vi "Calibration Utility.vi"() -> ()   [LabVIEW 2019]
panel:
  in  "Tab 1":enum32{"Page 1", "Page 2"}(tab)
  in  "Main Tab":T1(tab)
  in  "Tab 2":enum32{"Page 1", "Page 2"}(tab)
  out "Title":string="Calibration Utility, vBETA1"
  out "Date":string="2/21/2012"
  out "Time":string="2:11:48 PM"
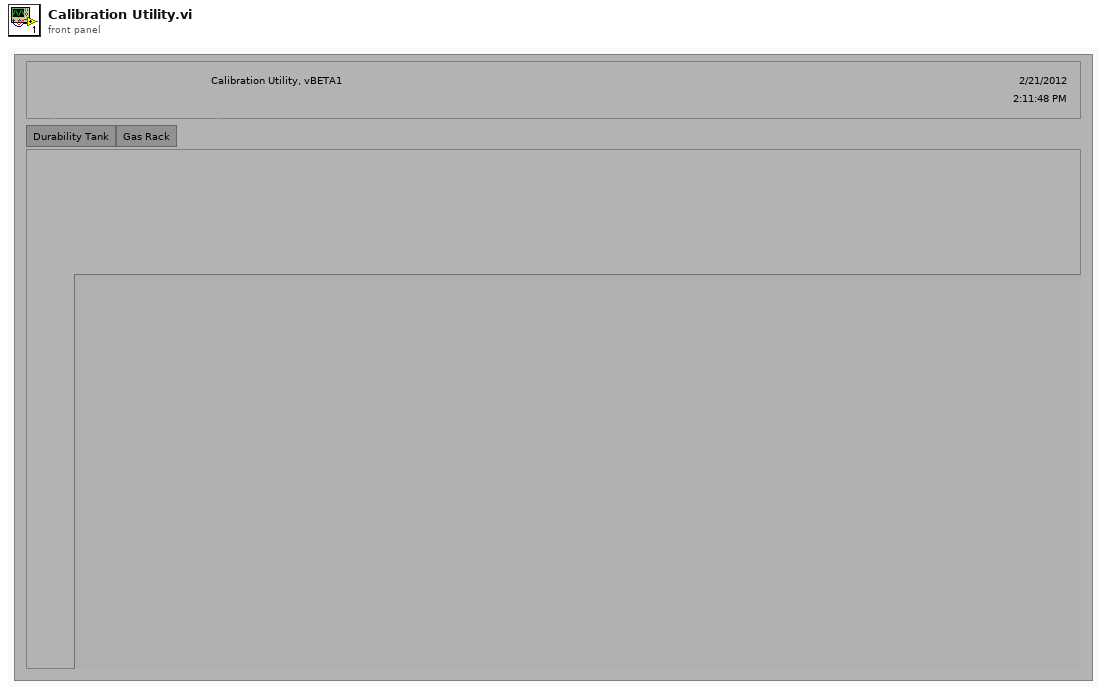
[diagram p1: front panel]
types:
  T1 = enum32{"Netway", "Durability Tank", "Gas Rack", "Dunk Tank"}
  T2 = enum32{"Page Enabled", "Page Disabled", "Page Disabled & Grayed"}
  T3 = enum32{"Invalid", "Standard", "Closed", "Hidden", "Minimized", "Maximized"}
  T4 = enum32{"invalid app kind", "Development System", "Run Time System", "Student Edition", "Embedded LabVIEW", "Evaluation", "Custom"}
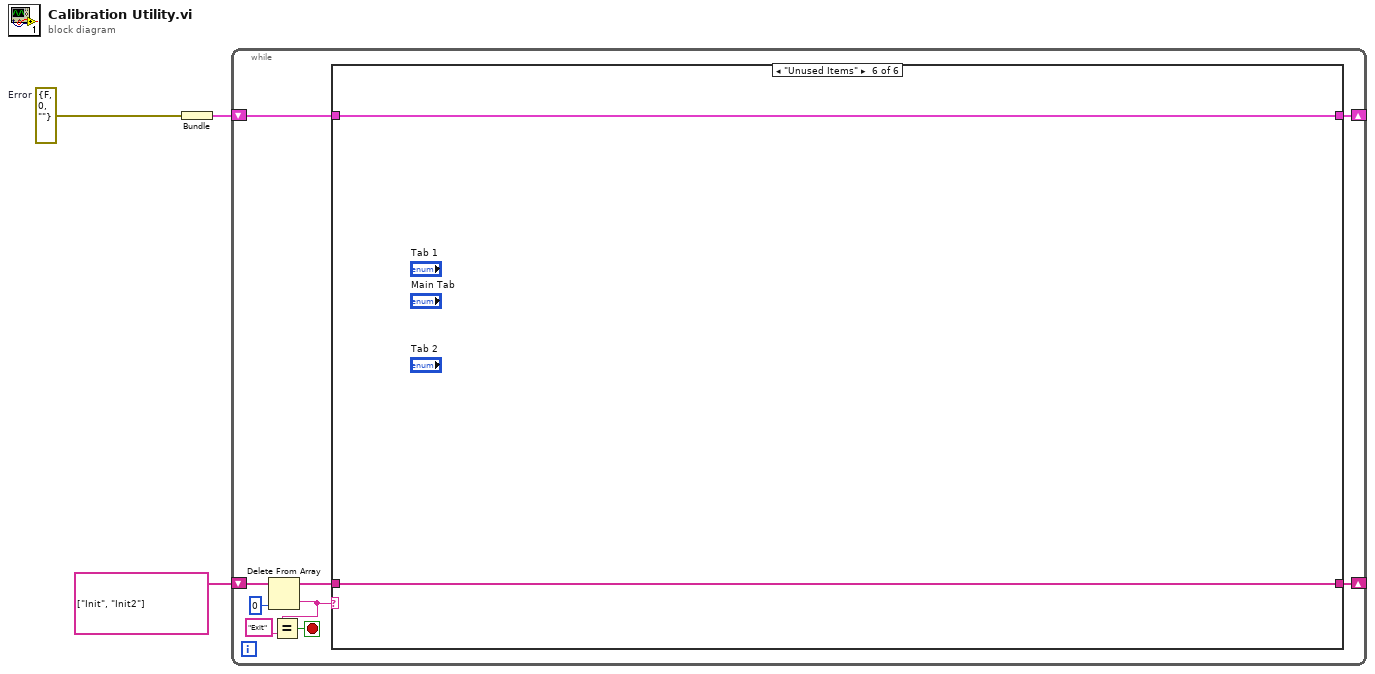
[diagram p0: block diagram]
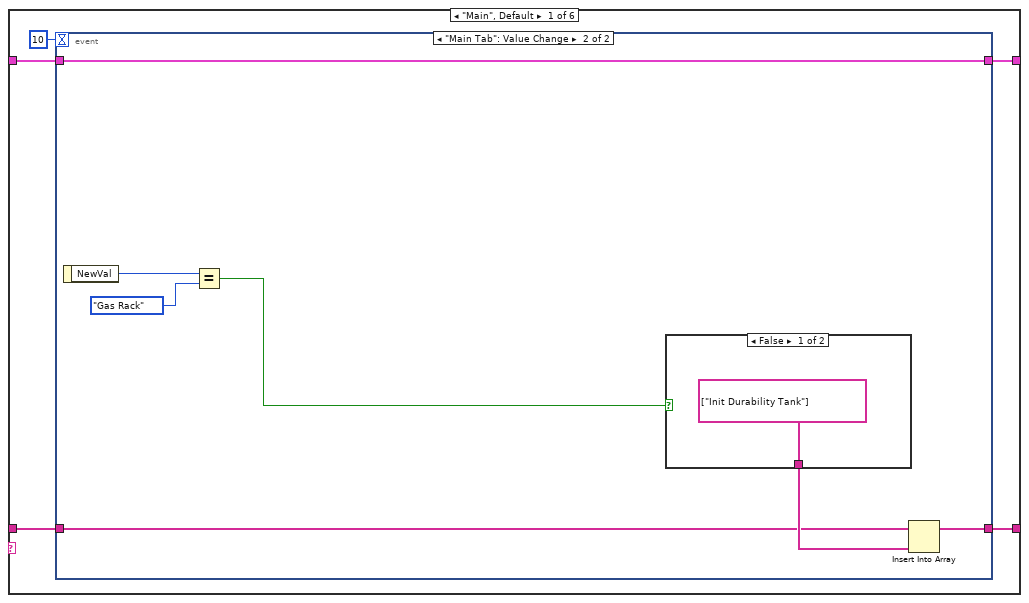
[diagram p2: hidden frame]
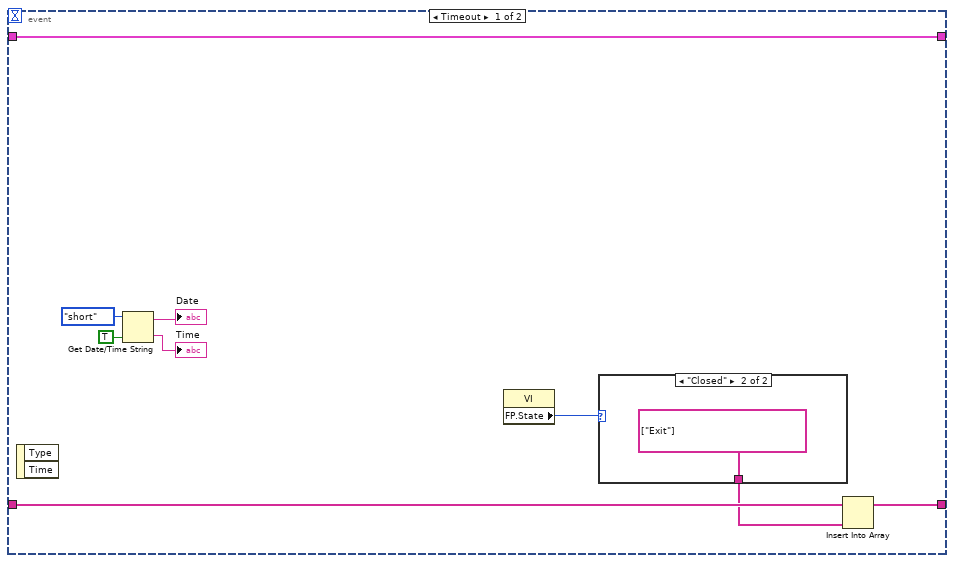
[diagram p3: hidden frame]
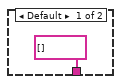
[diagram p4: hidden frame]
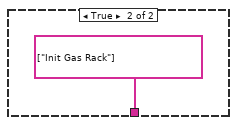
[diagram p5: hidden frame]
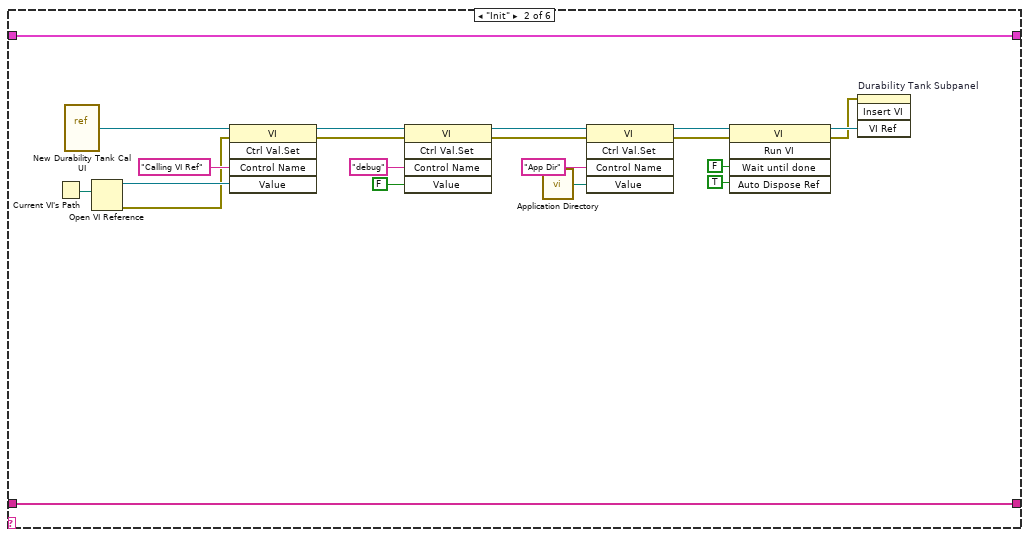
[diagram p6: hidden frame]
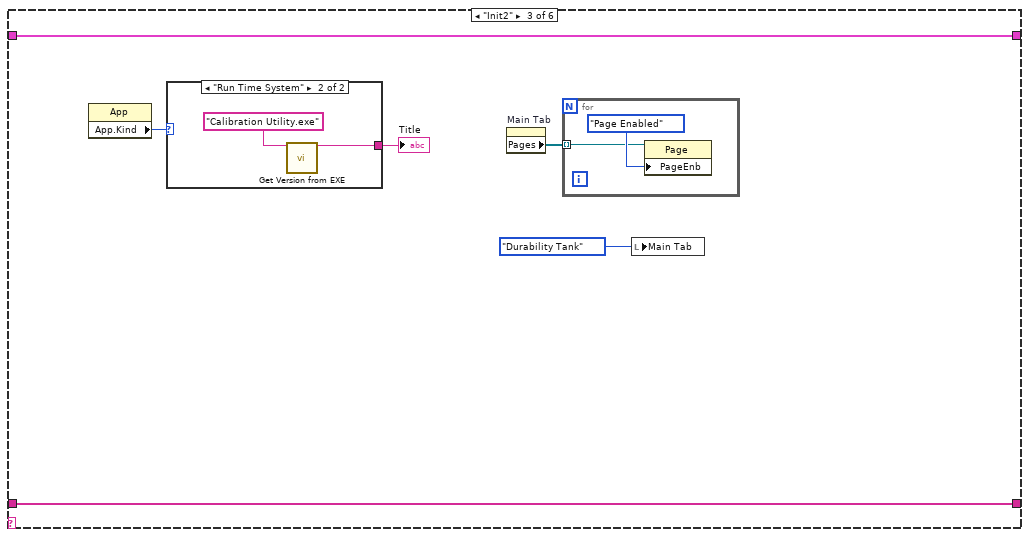
[diagram p7: hidden frame]
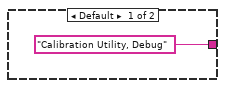
[diagram p8: hidden frame]
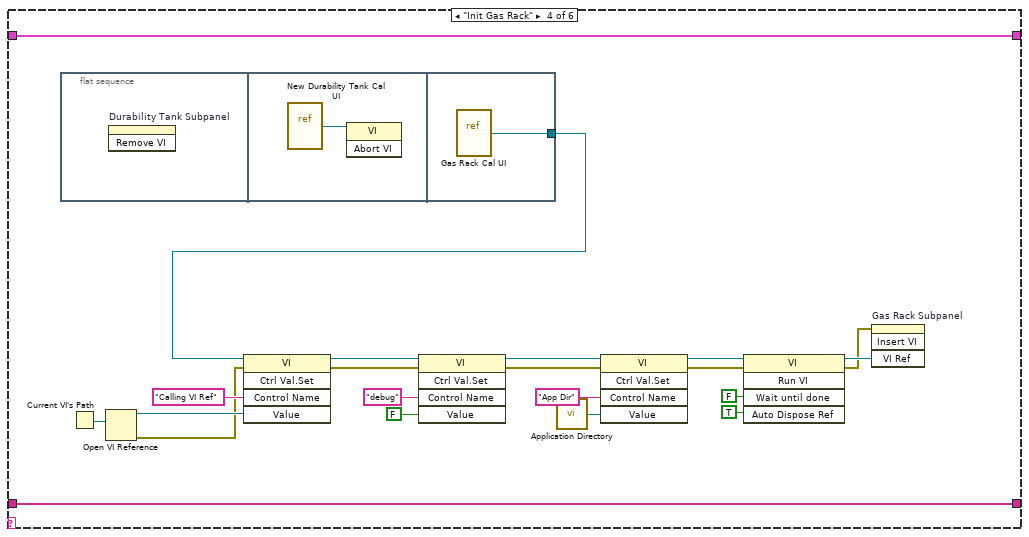
[diagram p9: hidden frame]
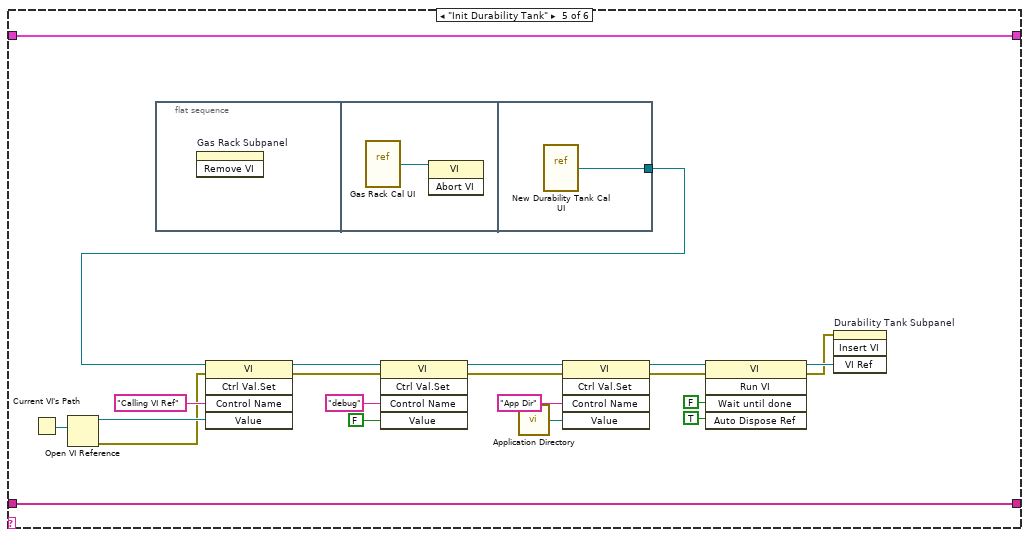
[diagram p10: hidden frame]
diagram:
  w1 = errorcluster {"status"=FALSE, "code"=0, "source"=""}  # Error
  n1 = Bundle("Error"=w1) -> (w2:cluster{"Error":errorcluster})  [unwired: 1 in]
  n2 = while {
    shift-right: [w9] -> _
    shift-left: string[] ["Init", "Init2"] -> [w12]
    shift-right: [w5] -> _
    shift-left: w2 -> [w6]
    stop <- w11 stop-if-true
    n3 = Delete From Array(array=w12, index=0) -> (deleted portion=w8:string, array with subset deleted=w10:string[])  [unwired: 1 in]
    n4 = Equal?(x=w8, y="Exit" ("x")) -> (x = y?=w11:bool)
    n5 = case shown="\"Unused Items\"" w8 {
      tunnel: [w15 w58 w63 w89 w112 w116] -> w9
      tunnel: w10 -> [w16 w58 w63 w89 w112 w116]
      tunnel: w6 -> [w14 w57 w64 w90 w113 w117]
      tunnel: [w13 w57 w64 w90 w113 w117] -> w5
      frame "Main", Default {
        n6 = event shown="[1] \"Main Tab\": Value Change" {
          selector: _ -> [_ _]
          dyn-events: _ -> [_ _]
          timeout: 10 -> [_ _]
          tunnel: [w21 w33] -> w15
          tunnel: w16 -> [w20 w32]
          tunnel: [w22 w35] -> w13
          tunnel: w14 -> [w22 w35]
          event Timeout {
            n7 = event-data() -> ()  [unwired: 1 in, 2 out]
            n8 = Get Date/Time String(date format (0)=enum16{"short", "long", "abbreviated"}."short", want seconds? (F)=TRUE) -> (date string=→"Date":string, time string=→"Time":string)  [unwired: 1 in]
            n9 = property class="VI"() -> ("FP.State"=w18:T3)  [unwired: 2 in, 2 out]
            n10 = case shown="\"Closed\"" w18 {
              tunnel: [string[] [] string[] ["Exit"]] -> w19
              frame Default {
              }
              frame "Closed" {
              }
            }
            n11 = Insert Into Array(array=w20, new element=w19) -> (w21:string[])  [unwired: 1 in]
          }
          event "Main Tab": Value Change {
            n12 = event-data() -> ("NewVal"=w30:T1)  [unwired: 1 in]
            n13 = Equal?(x=w30, y=T1."Gas Rack" ("x")) -> (x = y?=w31:bool)
            n14 = case shown="False" w31 {
              tunnel: [string[] ["Init Durability Tank"] string[] ["Init Gas Rack"]] -> w34
              frame False {
              }
              frame True {
              }
            }
            n15 = Insert Into Array(array=w32, new element=w34) -> (w33:string[])  [unwired: 1 in]
          }
        }
      }
      frame "Init" {
        n16 = Current VI's Path() -> (path=w53:path)
        n17 = vi-ref "New Durability Tank Cal UI.vi"() -> (w52:refnum<vi>)
        n18 = Open VI Reference(vi path=w53) -> (vi reference=w47:refnum<vi>, error out=w38:errorcluster)  [unwired: 5 in]
        n19 = invoke class="VI" method="Ctrl Val.Set"(reference=w52, error in=w38, "Control Name"="Calling VI Ref", "Value"=w47) -> (reference out=w51:refnum<vi>, error out=w42:errorcluster)  [unwired: 1 in, 3 out]
        n20 = invoke class="VI" method="Ctrl Val.Set"(reference=w51, error in=w42, "Control Name"="debug", "Value"=FALSE ("Wait Until Done")) -> (reference out=w50:refnum<vi>, error out=w41:errorcluster)  [unwired: 1 in, 3 out]
        n21 = call <vilib>:"Application Directory.vi"() -> ("Application Directory"=w43:path)
        n22 = invoke class="VI" method="Ctrl Val.Set"(reference=w50, error in=w41, "Control Name"="App Dir", "Value"=w43) -> (reference out=w49:refnum<vi>, error out=w40:errorcluster)  [unwired: 1 in, 3 out]
        n23 = invoke class="VI" method="Run VI"(reference=w49, error in=w40, "Wait until done"=FALSE ("Wait Until Done"), "Auto Dispose Ref"=TRUE ("Auto Dispose Reference")) -> (reference out=w54:refnum<vi>, error out=w39:errorcluster)  [unwired: 1 in, 3 out]
        n24 = invoke on="Durability Tank Subpanel" class="SubPnl" method="Insert VI"(error in=w39, "VI Ref"=w54) -> ()  [unwired: 2 in, 4 out]
      }
      frame "Init2" {
        n25 = property class="App"() -> ("App.Kind"=w61:T4)  [unwired: 2 in, 2 out]
        n26 = case shown="\"Run Time System\"" w61 {
          tunnel: ["Calibration Utility, Debug" ("Name and Version") w67] -> w60
          frame Default {
          }
          frame "Run Time System" {
            n27 = call "Get Version from EXE.vi"("EXE Name"="Calibration Utility.exe") -> ("Name and Version"=w67:string)  [unwired: 12 in, 2 out]
          }
        }
        "Title" <- w60
        n28 = property on="Main Tab" class="TabCtl (strict)"() -> ("Pages"=w62:refnum<vi>[])  [unwired: 2 in, 2 out]
        n29 = for {
          tunnel: w62 -> [w68] mode=indexing
          n30 = property class="Page"(reference=w68, "PageEnb"=T2."Page Enabled" ("Page Enabled State")) -> ()  [unwired: 1 in, 2 out]
        }
        n31 = local write "Main Tab"(T1."Durability Tank" ("Main Tab")) -> ()
      }
      frame "Init Gas Rack" {
        n32 = flat-sequence {
          tunnel: [w92] -> w70
          frame #0 {
            n33 = invoke on="Durability Tank Subpanel" class="SubPnl" method="Remove VI"() -> ()  [unwired: 3 in, 3 out]
          }
          frame #1 {
            n34 = vi-ref "New Durability Tank Cal UI.vi"() -> (w91:refnum<vi>)
            n35 = invoke class="VI" method="Abort VI"(reference=w91) -> ()  [unwired: 2 in, 3 out]
          }
          frame #2 {
            n36 = vi-ref "Gas Rack Cal UI.vi"() -> (w92:refnum<vi>)
          }
        }
        n37 = Current VI's Path() -> (path=w79:path)
        n38 = Open VI Reference(vi path=w79) -> (vi reference=w84:refnum<vi>, error out=w71:errorcluster)  [unwired: 5 in]
        n39 = invoke class="VI" method="Ctrl Val.Set"(reference=w70, error in=w71, "Control Name"="Calling VI Ref", "Value"=w84) -> (reference out=w80:refnum<vi>, error out=w75:errorcluster)  [unwired: 1 in, 3 out]
        n40 = invoke class="VI" method="Ctrl Val.Set"(reference=w80, error in=w75, "Control Name"="debug", "Value"=FALSE ("Wait Until Done")) -> (reference out=w81:refnum<vi>, error out=w74:errorcluster)  [unwired: 1 in, 3 out]
        n41 = call <vilib>:"Application Directory.vi"() -> ("Application Directory"=w88:path)
        n42 = invoke class="VI" method="Ctrl Val.Set"(reference=w81, error in=w74, "Control Name"="App Dir", "Value"=w88) -> (reference out=w82:refnum<vi>, error out=w73:errorcluster)  [unwired: 1 in, 3 out]
        n43 = invoke class="VI" method="Run VI"(reference=w82, error in=w73, "Wait until done"=FALSE ("Wait Until Done"), "Auto Dispose Ref"=TRUE ("Auto Dispose Reference")) -> (reference out=w76:refnum<vi>, error out=w72:errorcluster)  [unwired: 1 in, 3 out]
        n44 = invoke on="Gas Rack Subpanel" class="SubPnl" method="Insert VI"(error in=w72, "VI Ref"=w76) -> ()  [unwired: 2 in, 4 out]
      }
      frame "Init Durability Tank" {
        n45 = Current VI's Path() -> (path=w108:path)
        n46 = Open VI Reference(vi path=w108) -> (vi reference=w103:refnum<vi>, error out=w94:errorcluster)  [unwired: 5 in]
        n47 = flat-sequence {
          tunnel: [w115] -> w93
          frame #0 {
            n48 = invoke on="Gas Rack Subpanel" class="SubPnl" method="Remove VI"() -> ()  [unwired: 3 in, 3 out]
          }
          frame #1 {
            n49 = vi-ref "Gas Rack Cal UI.vi"() -> (w114:refnum<vi>)
            n50 = invoke class="VI" method="Abort VI"(reference=w114) -> ()  [unwired: 2 in, 3 out]
          }
          frame #2 {
            n51 = vi-ref "New Durability Tank Cal UI.vi"() -> (w115:refnum<vi>)
          }
        }
        n52 = invoke class="VI" method="Ctrl Val.Set"(reference=w93, error in=w94, "Control Name"="Calling VI Ref", "Value"=w103) -> (reference out=w107:refnum<vi>, error out=w98:errorcluster)  [unwired: 1 in, 3 out]
        n53 = invoke class="VI" method="Ctrl Val.Set"(reference=w107, error in=w98, "Control Name"="debug", "Value"=FALSE ("Wait Until Done")) -> (reference out=w106:refnum<vi>, error out=w97:errorcluster)  [unwired: 1 in, 3 out]
        n54 = call <vilib>:"Application Directory.vi"() -> ("Application Directory"=w99:path)
        n55 = invoke class="VI" method="Ctrl Val.Set"(reference=w106, error in=w97, "Control Name"="App Dir", "Value"=w99) -> (reference out=w105:refnum<vi>, error out=w96:errorcluster)  [unwired: 1 in, 3 out]
        n56 = invoke class="VI" method="Run VI"(reference=w105, error in=w96, "Wait until done"=FALSE ("Wait Until Done"), "Auto Dispose Ref"=TRUE ("Auto Dispose Reference")) -> (reference out=w109:refnum<vi>, error out=w95:errorcluster)  [unwired: 1 in, 3 out]
        n57 = invoke on="Durability Tank Subpanel" class="SubPnl" method="Insert VI"(error in=w95, "VI Ref"=w109) -> ()  [unwired: 2 in, 4 out]
      }
      frame "Unused Items" {
      }
    }
  }
